vi "Data Type Conversion FXP(+-,14,1) to FXP(+-,18,1)x8ch.vi"(4 "data in":T1={"channel 0"=[0.0, 0.0], "channel 1"=[0.0, 0.0], "channel 2"=[0.0, 0.0], "channel 3"=[0.0, 0.0], "channel 4"=[0.0, 0.0], "channel 5"=[0.0, 0.0], "channel 6"=[0.0, 0.0], "channel 7"=[0.0, 0.0]}) -> (0 "data out":T2, 1 "overflow":bool)   [LabVIEW 2015]
doc: "Converts data type from one format to another. The acceptable data types are: +- FXP 18,1; +-, FXP 14,1; and I16.\n\n<B>Supported data types</B>\nFXP +-,18,1; FXP +-,14,1; I16\n\n<B>Supported channel size</B>\n4, 8\n\n<B>Supported samples per cycle</B>\n2\n\n<B>Input Parameters</B>\n\n<B>data in</B> specifies the data to convert to another data type.\n\n<B>Output Parameters</B>\n\n<B>data out</B> returns the converted data.\n\n<B>overflow</B> returns the overflow carried through the data path."
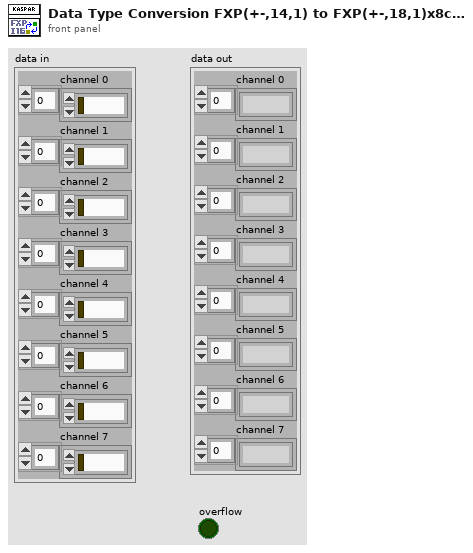
[diagram p1: front panel]
types:
  T1 = cluster{"channel 0":fxp<+/-,14,1>[], "channel 1":fxp<+/-,14,1>[], "channel 2":fxp<+/-,14,1>[], "channel 3":fxp<+/-,14,1>[], "channel 4":fxp<+/-,14,1>[], "channel 5":fxp<+/-,14,1>[], "channel 6":fxp<+/-,14,1>[], "channel 7":fxp<+/-,14,1>[]}
  T2 = cluster{"channel 0":fxp<+/-,18,1>[], "channel 1":fxp<+/-,18,1>[], "channel 2":fxp<+/-,18,1>[], "channel 3":fxp<+/-,18,1>[], "channel 4":fxp<+/-,18,1>[], "channel 5":fxp<+/-,18,1>[], "channel 6":fxp<+/-,18,1>[], "channel 7":fxp<+/-,18,1>[]}
  T3 = cluster{"data out":fxp<+/-,18,1>[], "data out":fxp<+/-,18,1>[], "data out":fxp<+/-,18,1>[], "data out":fxp<+/-,18,1>[], "data out":fxp<+/-,18,1>[], "data out":fxp<+/-,18,1>[], "data out":fxp<+/-,18,1>[], "data out":fxp<+/-,18,1>[]}
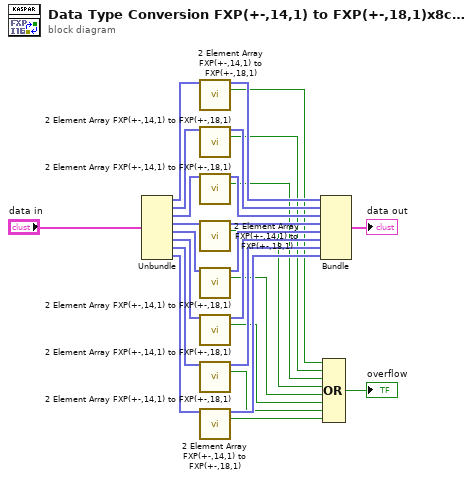
[diagram p0: block diagram]
diagram:
  n1 = Unbundle("data in") -> ("channel 0"=w27:fxp<+/-,14,1>[], "channel 1"=w25:fxp<+/-,14,1>[], "channel 2"=w23:fxp<+/-,14,1>[], "channel 3"=w21:fxp<+/-,14,1>[], "channel 4"=w19:fxp<+/-,14,1>[], "channel 5"=w13:fxp<+/-,14,1>[], "channel 6"=w15:fxp<+/-,14,1>[], "channel 7"=w17:fxp<+/-,14,1>[])
  n2 = call "2 Element Array FXP(+-,14,1) to FXP(+-,18,1).vi"("data in"=w27) -> ("data out"=w26:fxp<+/-,18,1>[], "overflow"=w9:bool)  [unwired: 13 in]
  n3 = call "2 Element Array FXP(+-,14,1) to FXP(+-,18,1).vi"("data in"=w25) -> ("data out"=w24:fxp<+/-,18,1>[], "overflow"=w8:bool)  [unwired: 13 in]
  n4 = call "2 Element Array FXP(+-,14,1) to FXP(+-,18,1).vi"("data in"=w23) -> ("data out"=w22:fxp<+/-,18,1>[], "overflow"=w7:bool)  [unwired: 13 in]
  n5 = call "2 Element Array FXP(+-,14,1) to FXP(+-,18,1).vi"("data in"=w21) -> ("data out"=w20:fxp<+/-,18,1>[], "overflow"=w6:bool)  [unwired: 13 in]
  n6 = call "2 Element Array FXP(+-,14,1) to FXP(+-,18,1).vi"("data in"=w19) -> ("data out"=w18:fxp<+/-,18,1>[], "overflow"=w5:bool)  [unwired: 13 in]
  n7 = call "2 Element Array FXP(+-,14,1) to FXP(+-,18,1).vi"("data in"=w13) -> ("data out"=w12:fxp<+/-,18,1>[], "overflow"=w4:bool)  [unwired: 13 in]
  n8 = call "2 Element Array FXP(+-,14,1) to FXP(+-,18,1).vi"("data in"=w15) -> ("data out"=w14:fxp<+/-,18,1>[], "overflow"=w3:bool)  [unwired: 13 in]
  n9 = call "2 Element Array FXP(+-,14,1) to FXP(+-,18,1).vi"("data in"=w17) -> ("data out"=w16:fxp<+/-,18,1>[], "overflow"=w2:bool)  [unwired: 13 in]
  n10 = Bundle("data out"=w26, "data out"=w24, "data out"=w22, "data out"=w20, "data out"=w18, "data out"=w12, "data out"=w14, "data out"=w16) -> (→"data out":T3)  [unwired: 1 in]
  n11 = Compound Arithmetic op=OR(w9, w8, w7, w6, w5, w4, w3, w2) -> (→"overflow":bool)
